vi "DigitalINRead.vi"(8 "error in (no error)":errorcluster caption="错误输入（无错误）", 10 "size":i32=2048, 11 "handle":u64) -> (0 "error out":errorcluster caption="错误输出", 1 "RxBuffer out":u16[](array[numeric]), 2 "function return":i32, 3 "handle out":u64, 5 "backsize out":i32)   [LabVIEW 2018]
doc: "Set pos. or neg. Supply voltage"
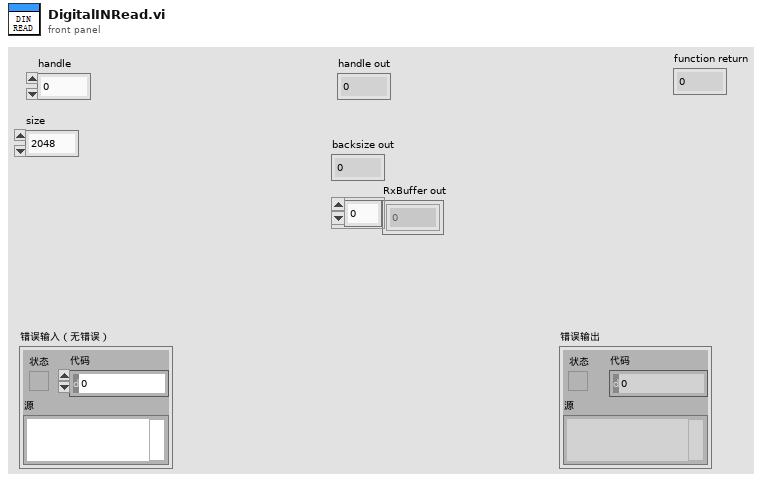
[diagram p1: front panel]
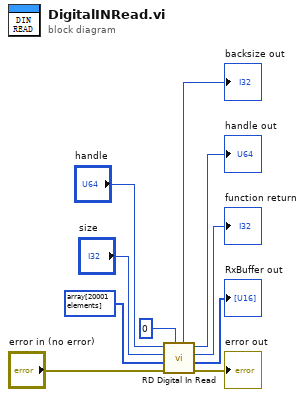
[diagram p0: block diagram]
diagram:
  n1 = call "RD Digital In Read.vi"("backsize"=0, "error in (no error)"="error in (no error)", "RxBuffer"=u16[] array[20001 elements], "size"="size", "handle"="handle") -> ("error out"=→"error out":errorcluster, "RxBuffer out"=→"RxBuffer out":u16[], "function return"=→"function return":i32, "handle out"=→"handle out":u64, "backsize out"=→"backsize out":i32)  [unwired: 2 in]
